vi "PC main.vi"() -> ()   [LabVIEW 2021]
uses:
  Force waveform.ctl
  PID gain.ctl
panel:
  in  "PID gains":T1={"proportional gain (Kc)"=0.1, "integral time (Ti, min)"=0.12, "derivative time (Td, min)"=0.0} {"derivative time (Td, min)" format="%.3f"; "integral time (Ti, min)" format="%.3f"; "proportional gain (Kc)" format="%.3f"}
  out "FF predict":dbl
  out "Input Voltage":dbl
  in  "FF_gain":dbl(slide)=1.0 scale=0.0..3.0
  out "Waveform Chart":cluster{"Mes force":dbl, "Ref force":dbl}(graph)
  in  "Ref force":dbl(slide) scale=0.0..120.0
  in  "PID ON/OFF":bool
  in  "record start":bool
  in  "Stop \"PC Main\"":bool
  in  "Stop \"Motor control\"":bool
  in  "Motor enable":bool
  # "Single Motor Force Control"
  # "INITIALIZE"
  # "PID TUNE"
  # "STOP"
  # "RECORD"
  # "FEED FORWARD TUNE"
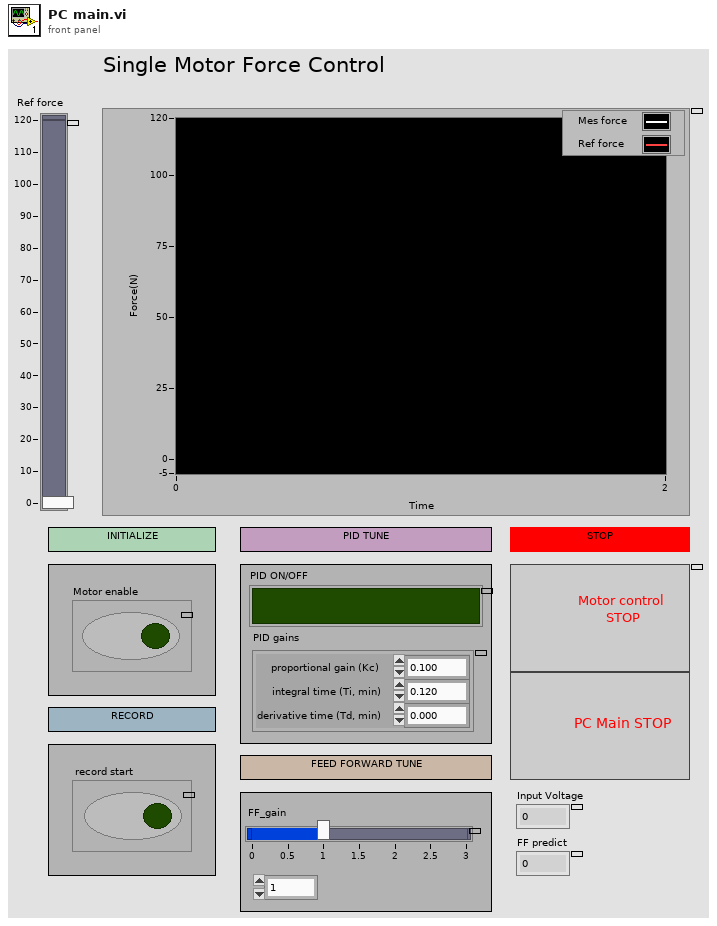
[diagram p1: front panel]
types:
  T1 = typedef "PID gain.ctl" = cluster{"proportional gain (Kc)":dbl, "integral time (Ti, min)":dbl, "derivative time (Td, min)":dbl}
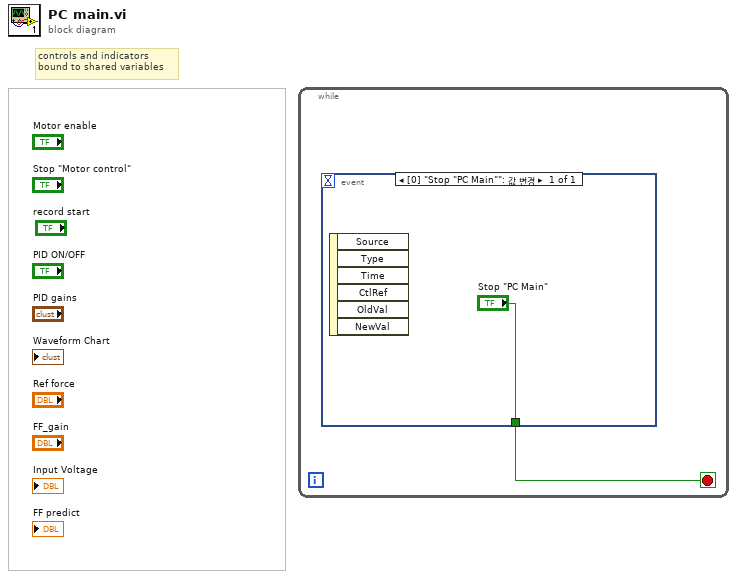
[diagram p0: block diagram]
diagram:
  # "controls and indicators\nbound to shared variables"
  n1 = while {
    stop <- w1 stop-if-true
    n2 = event shown="[0] \"Stop \"PC Main\"\": 값 변경" {
      selector: _ -> [_]
      dyn-events: _ -> [_]
      timeout: _ -> [_]
      tunnel: ["Stop \"PC Main\""] -> w1
      event "Stop \"PC Main\"": Value Change {
        n3 = event-data() -> ()  [unwired: 1 in, 6 out]
      }
    }
  }
